vi "Registration Confirmation.vi"(8 "error in":errorcluster) -> (0 "error out":errorcluster)   [LabVIEW 2015, in "Generic Module Library.lvlib" / "Template G_Module.lvlib"]
uses:
  Template G_Module.lvlib
  Private API/Module Broadcasts/Broadcast Support/Registration Actions.ctl
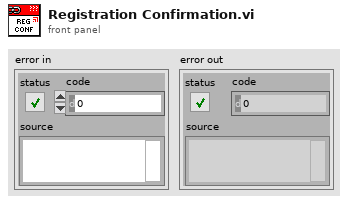
[diagram p1: front panel]
types:
  T1 = typedef "Generic Module Library.lvlib/Template G_Module.lvlib/Registration Actions.ctl" = enum16{"Create", "Get", "Destroy"}
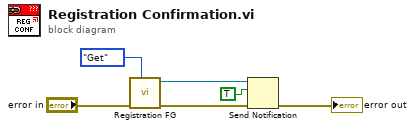
[diagram p0: block diagram]
diagram:
  n1 = call "Registration FG.vi"("Registration Actions"=Registration_Actions."Get", "error in"="error in") -> ("error out"=w4:errorcluster, "notifier out"=w3:refnum<notifier>)  [unwired: 8 in]
  n2 = Send Notification(notification=TRUE, notifier=w3, error in (no error)=w4) -> (error out=→"error out":errorcluster)  [unwired: 1 out]
